vi "Initialize.vi"(7 "Serial Configuration":T1={"Baud Rate"=9600, "Parity"=0, "Data Bits"=8, "Stop Bits"=10, "Flow Control"=0} {"Flow Control" items=["None", "XON/XOFF", "RTS/CTS", "XON/XOFF & RTS/CTS", "DTR/DSR", "XON/XOFF & DTR/DSR"]; "Stop Bits" items=["1.0"=10, "1.5"=15, "2.0"=20]; "Data Bits" items=["7"=7, "8"=8]; "Parity" items=["None", "Odd", "Even", "Mark", "Space"]; "Baud Rate" items=["300"=300, "600"=600, "1200"=1200, "2400"=2400, "4800"=4800, "9600"=9600, "19200"=19200]}, 8 "error in (no error)":errorcluster, 9 "Reset (True)":bool=TRUE, 10 "ID Query (True)":bool=TRUE, 11 "VISA resource name":refnum<visa-resource-name>) -> (0 "error out":errorcluster, 3 "VISA resource name out":refnum<visa-resource-name>)   [LabVIEW 2020, in "IT6500.lvlib"]
doc: "Establishes communication with the instrument and optionally performs an instrument identification query and/or an instrument reset. It also places the instrument in a default state needed for other instrument driver operations. Therefore, call this VI before calling other instrument driver VIs for this instrument. Generally, you need to call the <b>Initialize</b> VI only once at the beginning of an application."
uses:
  IT6500.lvlib
panel:
  # "(c) 2014 <Enter Company Name Here>.  ALL RIGHTS RESERVED."
  # "EDIT: Change control description to remove example text for buses not supported."
  # "EDIT: Serial settings must match those on the physical instrument.  Review user's manual to determine the correct Flow Control protocol for the instrument.  \"None\" is the least robust option for this setting, and could lead to unreliable data transmission."
  # "EDIT: If your instrument does not support ID query or Reset, remove the ID Query or Reset control from the front panel and delete the case structure with the ID Query or Reset code from the block diagram."
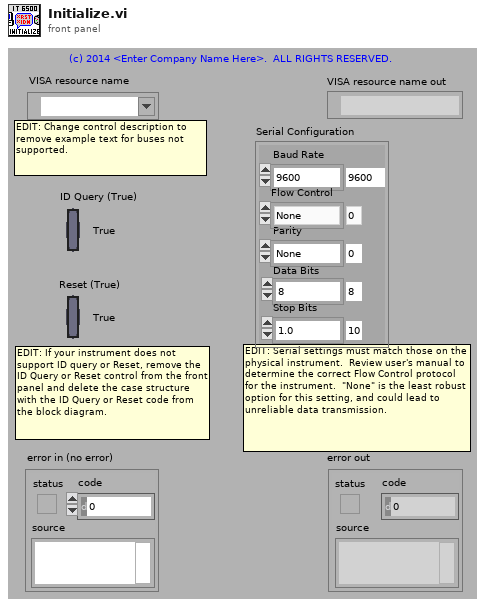
[diagram p1: front panel]
types:
  T1 = cluster{"Baud Rate":u32, "Parity":u16, "Data Bits":u16, "Stop Bits":u16, "Flow Control":u16}
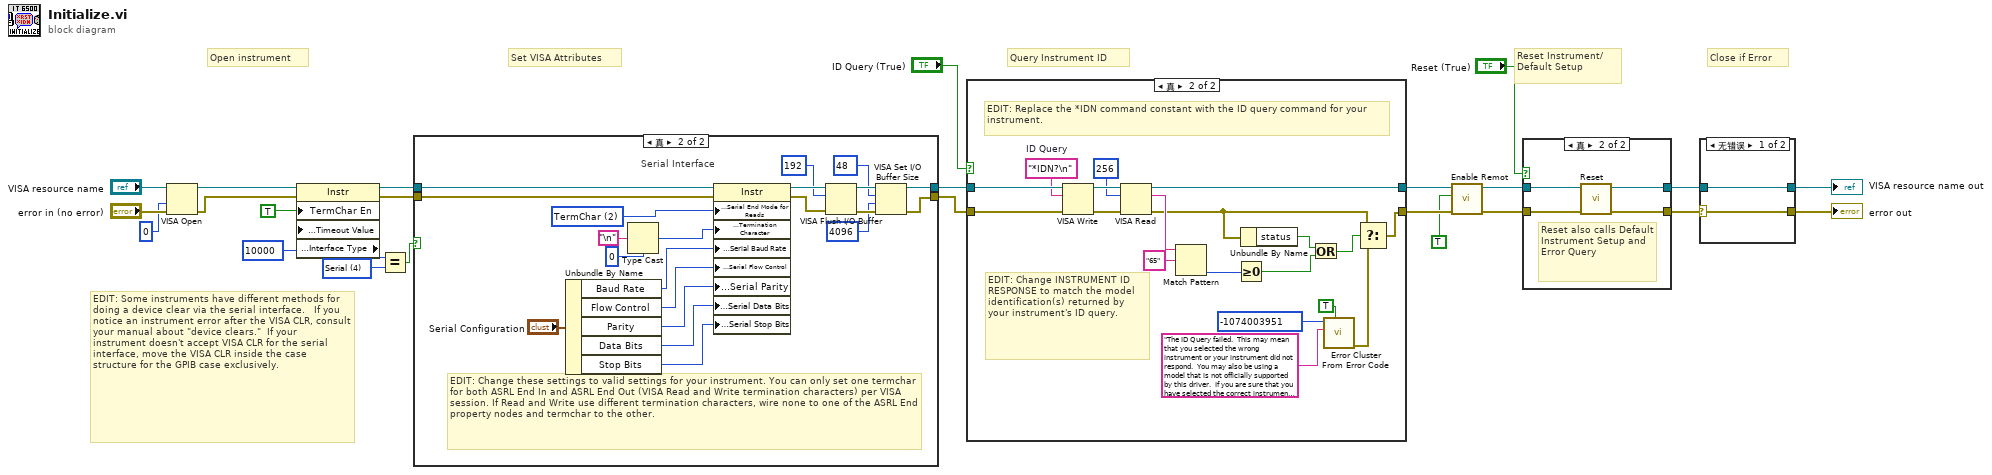
[diagram p0: block diagram]
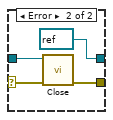
[diagram p3: hidden frame]
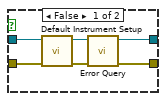
[diagram p4: hidden frame]
diagram:
  w14 = u16 4 items=["GPIB"=1, "VXI"=2, "GPIB-VXI"=3, "Serial"=4, "PXI"=5, "TCPIP"=6, "USB"=7] ("Interface Information:Interface Type")
  # "EDIT: Some instruments have different methods for doing a device clear via the serial interface.   If you notice an instrument error after the VISA CLR, consult your manual about \"device clears.\"  If your instrument doesn't accept VISA CLR for the serial interface, move the VISA CLR inside the case  structure for the GPIB case exclusively."
  # "Set VISA Attributes"
  # "Close if Error"
  # "Query Instrument ID"
  # "Reset Instrument/\nDefault Setup"
  # "Open instrument"
  n1 = VISA Open(access mode=u32 0, error in (no error)="error in (no error)", VISA resource name="VISA resource name") -> (VISA resource name=w12:refnum<visa-resource-name>, error out=w11:errorcluster)  [unwired: 2 in]
  n2 = property class="Instr"(reference=w12, error in=w11, "TermChar En"=TRUE, "General Settings:Timeout Value"=u32 10000) -> (reference out=w17:refnum<visa-resource-name>, error out=w16:errorcluster, "Interface Information:Interface Type"=w21:u16)
  n3 = Equal?(x=w21, y=w14) -> (x = y?=w15:bool)
  n4 = case shown="真" w15 {
    tunnel: [w26 w45] -> w19
    tunnel: [w27 w42] -> w18
    tunnel: w17 -> [w26 w47]
    tunnel: w16 -> [w27 w48]
    frame False {
      # "EDIT: Remove interfaces not supported by your instrument."
      # "GPIB, TCP/IP, and USB Interface"
    }
    frame True {
      w28 = u16 2 items=["None", "LastBit", "TermChar"] ("Serial Settings:Serial End Mode for Reads")
      # "EDIT: Change these settings to valid settings for your instrument. You can only set one termchar for both ASRL End In and ASRL End Out (VISA Read and Write termination characters) per VISA session. If Read and Write use different termination characters, wire none to one of the ASRL End property nodes and termchar to the other."
      # "Serial Interface"
      n5 = Unbundle By Name("Serial Configuration") -> ("Baud Rate"=w34:u32, "Flow Control"=w30:u16, "Parity"=w32:u16, "Data Bits"=w33:u16, "Stop Bits"=w29:u16)
      n6 = Type Cast(type=u8 0, x="\n" ("Line Feed Constant")) -> (*(type *) &x=w35:u8)
      n7 = property class="Instr"(reference=w47, error in=w48, "Serial Settings:Serial End Mode for Reads"=w28, "Message Based Settings:Termination Character"=w35, "Serial Settings:Serial Baud Rate"=w34, "Serial Settings:Serial Flow Control"=w30, "Serial Settings:Serial Parity"=w32, "Serial Settings:Serial Data Bits"=w33, "Serial Settings:Serial Stop Bits"=w29) -> (reference out=w41:refnum<visa-resource-name>, error out=w44:errorcluster)
      n8 = VISA Flush I/O Buffer(VISA resource name=w41, mask (16)=u16 192, error in (no error)=w44) -> (VISA resource name out=w46:refnum<visa-resource-name>, error out=w43:errorcluster)
      n9 = VISA Set I/O Buffer Size(VISA resource name=w46, mask (16)=u16 48, size (4096)=u32 4096 ("size (0)"), error in (no error)=w43) -> (VISA resource name out=w45:refnum<visa-resource-name>, error out=w42:errorcluster)
    }
  }
  n10 = case shown="真" "ID Query (True)" {
    tunnel: [w49 w69] -> w4
    tunnel: [w50 w66] -> w5
    tunnel: w19 -> [w50 w67]
    tunnel: w18 -> [w49 w68]
    frame False {
    }
    frame True {
      w60 = "*IDN?\n"  # ID Query
      # "EDIT: Replace the *IDN command constant with the ID query command for your instrument."
      # "EDIT: Change INSTRUMENT ID RESPONSE to match the model identification(s) returned by your instrument's ID query."
      n11 = VISA Write(VISA resource name=w67, write buffer=w60, error in (no error)=w68) -> (VISA resource name out=w64:refnum<visa-resource-name>, error out=w63:errorcluster)  [unwired: 1 out]
      n12 = VISA Read(VISA resource name=w64, byte count=u32 256, error in (no error)=w63) -> (VISA resource name out=w66:refnum<visa-resource-name>, read buffer=w65:string, error out=w54:errorcluster)  [unwired: 1 out]
      n13 = Match Pattern(string=w65, regular expression="65") -> (offset past match=w55:i32)  [unwired: 1 in, 3 out]
      n14 = Greater Or Equal To 0?(x=w55) -> (x >= 0?=w52:bool)
      n15 = Unbundle By Name(w54) -> ("status"=w53:bool)
      n16 = Or(x=w53, y=w52) -> (x .or. y?=w51:bool)
      n17 = call <vilib>:"Error Cluster From Error Code.vi"("show call chain? (False)"=TRUE, "error message (\"\")"="The ID Query failed.  This may mean that you selected the wrong instrument or your instrument did not respond.  You may also be using a model that is not officially supported by this driver.  If you are sure that you have selected the correct instrument and it is responding, try disabling the ID Query." ("Source (VI Name)"), "error code (0)"=-1074003951 ("Code")) -> ("error out"=w59:errorcluster)  [unwired: 6 in]
      n18 = Select(t=w54, s=w51, f=w59) -> (s? t:f=w69:errorcluster)
    }
  }
  n19 = call "Enable Remot.vi"("error in (no error)"=w4, "Enable"=TRUE, "VISA resource name"=w5) -> ("error out"=w2:errorcluster, "VISA resource name out"=w3:refnum<visa-resource-name>)  [unwired: 7 in]
  n20 = case shown="真" "Reset (True)" {
    tunnel: w2 -> [w74 w76]
    tunnel: [w71 w79] -> w7
    tunnel: w3 -> [w75 w77]
    tunnel: [w72 w78] -> w8
    frame False {
      n21 = call "Default Instrument Setup.vi"("error in (no error)"=w74, "VISA resource name"=w75) -> ("error out"=w70:errorcluster, "VISA resource name out"=w73:refnum<visa-resource-name>)  [unwired: 8 in]
      n22 = call "Error Query.vi"("error in (no error)"=w70, "VISA resource name"=w73) -> ("error out"=w71:errorcluster, "VISA resource name out"=w72:refnum<visa-resource-name>)  [unwired: 6 in, 2 out]
    }
    frame True {
      # "Reset also calls Default Instrument Setup and Error Query"
      n23 = call "Reset.vi"("error in (no error)"=w76, "VISA resource name"=w77) -> ("error out"=w79:errorcluster, "VISA resource name out"=w78:refnum<visa-resource-name>)  [unwired: 8 in]
    }
  }
  n24 = case shown="无错误" w7 {
    selector: w7 -> [w80 w83]
    tunnel: w8 -> [w81 w84]
    tunnel: [w81 refnum<visa-resource-name> refnum ("VISA resource name out")] -> w10
    tunnel: [w80 w85] -> w9
    frame No Error {
    }
    frame Error {
      n25 = call "Close.vi"("error in (no error)"=w83, "VISA resource name"=w84) -> ("error out"=w85:errorcluster)  [unwired: 9 in]
    }
  }
  "VISA resource name out" <- w10
  "error out" <- w9
